vi "Configure UART.vi"(4 "RX GPIO":T1=17, 5 "Purpose (\"UART\")":string="UART", 6 "TX GPIO":T1=16, 7 "UART #":T2, 8 "error in (no error)":errorcluster, 9 "Term Char (None)":string, 10 "Baud":u32=115200, 11 "Session in":refnum<class "Session.lvclass">) -> (0 "error out":errorcluster, 3 "Session out":refnum<class "Session.lvclass">)   [LabVIEW 2024, in "CTI.lvlib" / "Session.lvclass"]
doc: "UARTs are simple asynchronous communication busses that are typically used for slower communications and legacy devices. With CTI, UARTs can be used in ASCII line mode by specifying the line-ending character (usually a newline '\\n'). If a Term Char is not specified then the UART will operate in binary mode."
uses:
  Session.lvclass
  UART Number.ctl
  GPIO Number.ctl
  UART Pins.ctl
  Session.lvclass/Session.ctl
  5d41f6f2-78eb-42d5-8031-5b57c1ee8460.vi
  Is Full Errors.vi
  Check Errors.vi
  CTI.lvlib
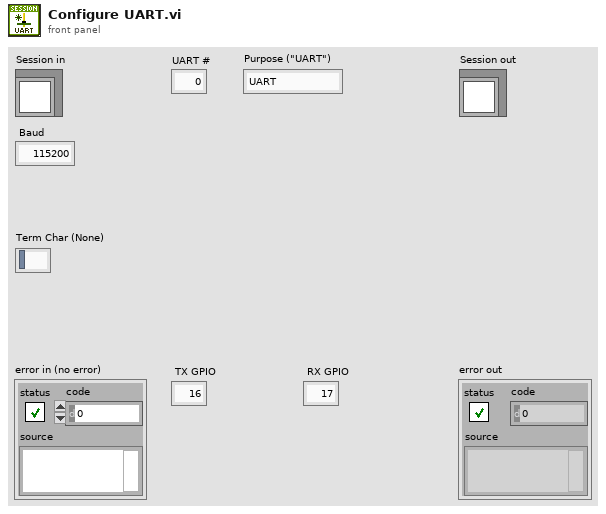
[diagram p1: front panel]
types:
  T1 = typedef "CTI.lvlib/GPIO Number.ctl" = i8
  T2 = typedef "CTI.lvlib/UART Number.ctl" = i8
  T3 = typedef "CTI.lvlib/UART Pins.ctl" = cluster{"TX GPIO":T1, "RX GPIO":T1}
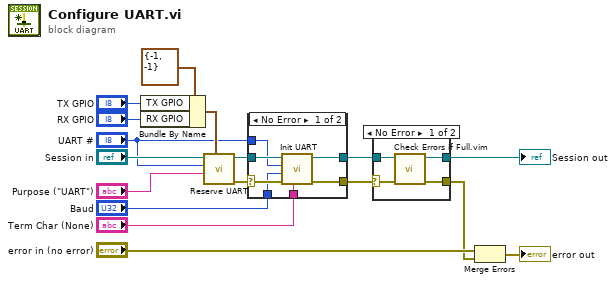
[diagram p0: block diagram]
diagram:
  n1 = Bundle By Name(cluster=T3 {"TX GPIO"=-1, "RX GPIO"=-1} ("UART Pins"), "TX GPIO"="TX GPIO", "RX GPIO"="RX GPIO") -> (w14:T3)
  n2 = call "Reserve UART.vi"("UART Pins"=w14, "Purpose"="Purpose (\"UART\")", "UART #"="UART #", "Session in"="Session in") -> ("error out"=w10:errorcluster, "Session out"=w9:refnum<class "Session.lvclass">)  [unwired: 6 in]
  n3 = case shown="No Error" w10 {
    selector: w10 -> [w23 w25]
    tunnel: w9 -> [w24 w26]
    tunnel: "Baud" -> [w22 _]
    tunnel: "Term Char (None)" -> [w21 _]
    tunnel: [w20 w26] -> w5
    tunnel: [w19 w25] -> w6
    tunnel: "UART #" -> [w18 _]
    frame No Error {
      n4 = call "Init UART.vi"("Term Char"=w21, "error in (no error)"=w23, "Baud"=w22, "UART In"=w18, "Session in"=w24) -> ("error out"=w19:errorcluster, "Session out"=w20:refnum<class "Session.lvclass">)  [unwired: 5 in]
    }
    frame Error {
    }
  }
  n5 = case shown="No Error" w6 {
    selector: w6 -> [w29 w31]
    tunnel: w5 -> [w30 w32]
    tunnel: [w28 w32] -> w4
    tunnel: [w27 w31] -> w2
    frame No Error {
      n6 = call "Check Errors if Full.vim"("error in (no error)"=w29, "Session in"=w30) -> ("error out"=w27:errorcluster, "Session out"=w28:refnum<class "Session.lvclass">)  [unwired: 8 in]
    }
    frame Error {
    }
  }
  "Session out" <- w4
  n7 = Merge Errors("error in (no error)", w2) -> (→"error out":errorcluster)
